vi "ReadCh1.vi"() -> ()   [LabVIEW 2014]
uses:
  <vilib>/DAQmx/create/channels.llb/DAQmx Create Channel (AI-Voltage-Basic).vi
  <vilib>/DAQmx/configure/timing.llb/DAQmx Timing (Sample Clock).vi
  <vilib>/DAQmx/read.llb/DAQmx Read (Analog Wfm 1Chan NSamp).vi
panel:
  in  "stop":bool
  out "Waveform Chart":waveform(dbl)(graph)
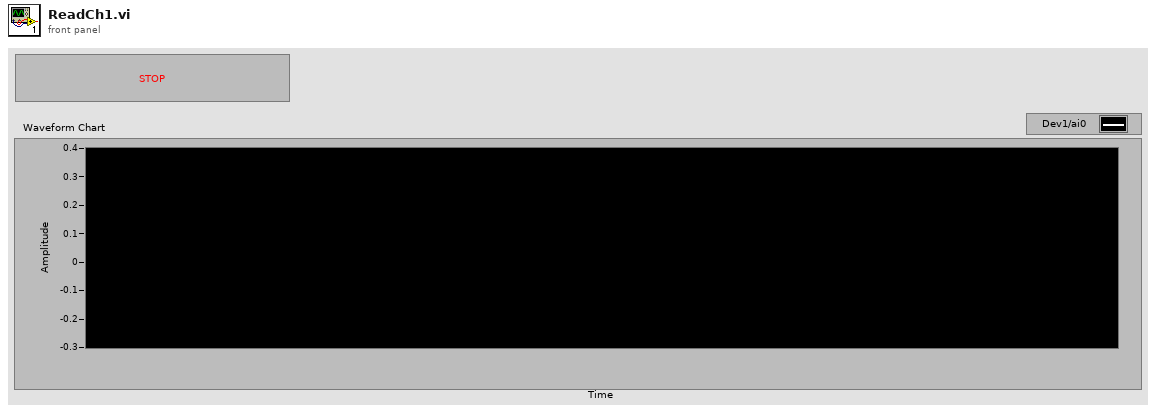
[diagram p1: front panel]
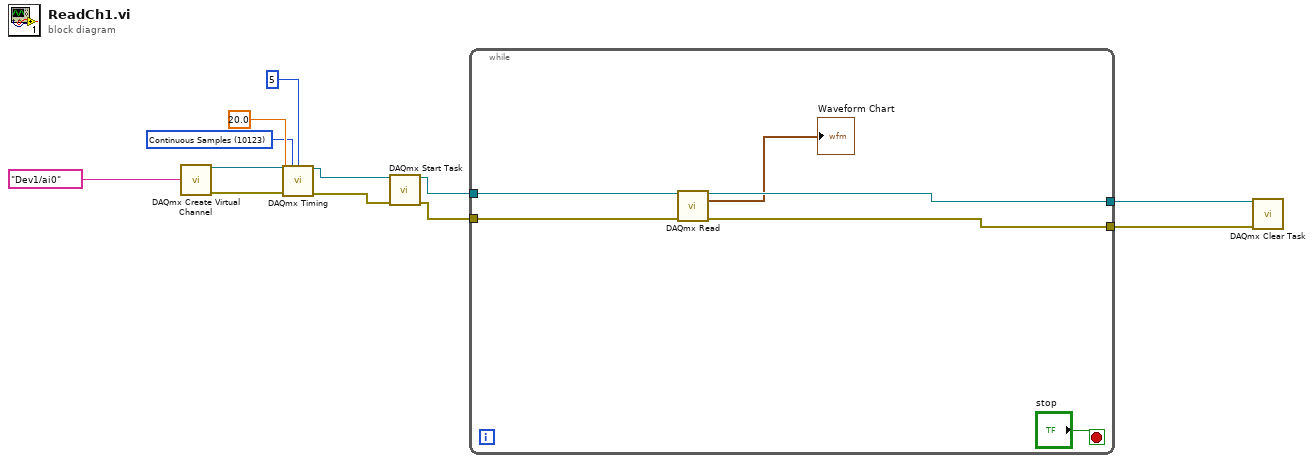
[diagram p0: block diagram]
diagram:
  w2 = 10123 items=["Finite Samples"=10178, "Continuous Samples"=10123, "Hardware Timed Single Point"=12522] ("sample mode")
  n1 = call-poly <vilib>:"DAQmx Create Virtual Channel.vi"("physical channels"=tag "Dev1/ai0") -> ("task out"=w8:refnum<k21>, "error out"=w12:errorcluster)  [unwired: 13 in]
  n2 = call-poly <vilib>:"DAQmx Timing.vi"("task/channels in"=w8, "sample mode"=w2, "samples per channel"=5, "rate"=20.0, "error in"=w12) -> ("task out"=w7:refnum<k21>, "error out"=w11:errorcluster)  [unwired: 9 in]
  n3 = call <vilib>:"DAQmx Start Task.vi"("task/channels in"=w7, "error in"=w11) -> ("task out"=w6:refnum<k21>, "error out"=w10:errorcluster)  [unwired: 12 in]
  n4 = while {
    tunnel: w10 -> [w18]
    tunnel: [w17] -> w9
    tunnel: w6 -> [w16]
    tunnel: [w15] -> w5
    stop <- "stop" stop-if-true
    n5 = call-poly <vilib>:"DAQmx Read.vi"("task/channels in"=w16, "error in"=w18) -> ("task out"=w15:refnum<k21>, "data"=→"Waveform Chart":waveform(dbl), "error out"=w17:errorcluster)  [unwired: 11 in]
  }
  n6 = call <vilib>:"DAQmx Clear Task.vi"("task in"=w5, "error in"=w9) -> ()  [unwired: 13 in, 1 out]
